vi "G#Object_CastFromLabVIEWObject.vi"(5 "LabVIEWObject in":refnum<class>) -> (0 "is of G#Object?":bool, 1 "not a refnum?":bool, 2 "reference out":refnum<class "G#Object.lvclass">)   [LabVIEW 2017, in "G#Object.lvclass"]
doc: "Cast from a native LabVIEW object reference to a G#Object reference."
uses:
  G#Object.lvclass
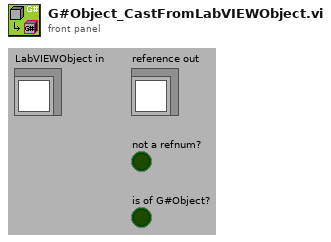
[diagram p1: front panel]
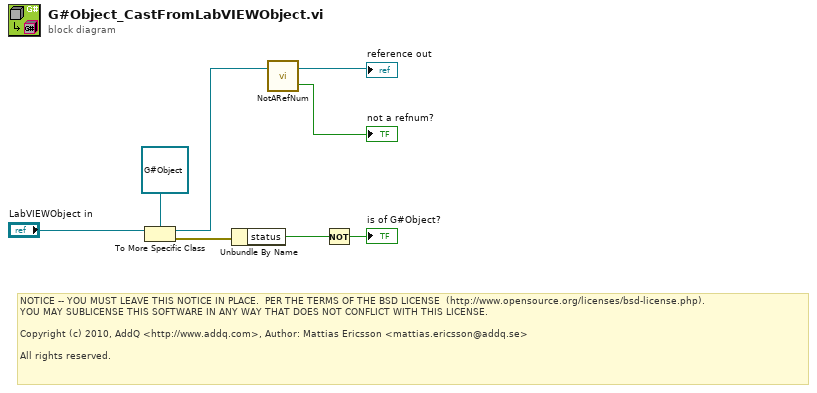
[diagram p0: block diagram]
diagram:
  # "NOTICE -- YOU MUST LEAVE THIS NOTICE IN PLACE.  PER THE TERMS OF THE BSD LICENSE  (http://www.opensource.org/licenses/bsd-license.php).\nYOU MAY SUBLICENSE THIS SOFTWARE IN ANY WAY THAT DOES NOT CONFLICT WITH THIS LICENSE.\n\nCopyright (c) 2010, AddQ <http://www.addq.com>, Author: Mattias Ericsson <mattias.ericsson@addq.se>\n\nAll rights reserved."
  n1 = To More Specific Class(target class=refnum<class "G#Object.lvclass"> refnum ("G#Object.lvclass"), reference="LabVIEWObject in") -> (specific class reference=w3:refnum<class "G#Object.lvclass">, error out=w8:errorcluster)  [unwired: 1 in]
  n2 = Unbundle By Name(w8) -> ("status"=w7:bool)
  n3 = call-dynamic "NotARefNum.vi"("reference in"=w3) -> ("not a refnum?"=→"not a refnum?":bool, "reference out"=→"reference out":refnum<class "G#Object.lvclass">)  [unwired: 1 in]
  n4 = Not(x=w7) -> (.not. x?=→"is of G#Object?":bool)
